vi "Test_AddMeas.vi"() -> ()   [LabVIEW 2019]
uses:
  ByteGSAPIBase.lvclass
panel:
  in  "ByteGSAPIBase in":refnum<class "ByteGSAPIBase.lvclass">
  out "ByteGSAPIBase out":refnum<class "ByteGSAPIBase.lvclass">
  out "Measurement_Id":i32
  out "error out":errorcluster
  in  "error in (no error)":errorcluster
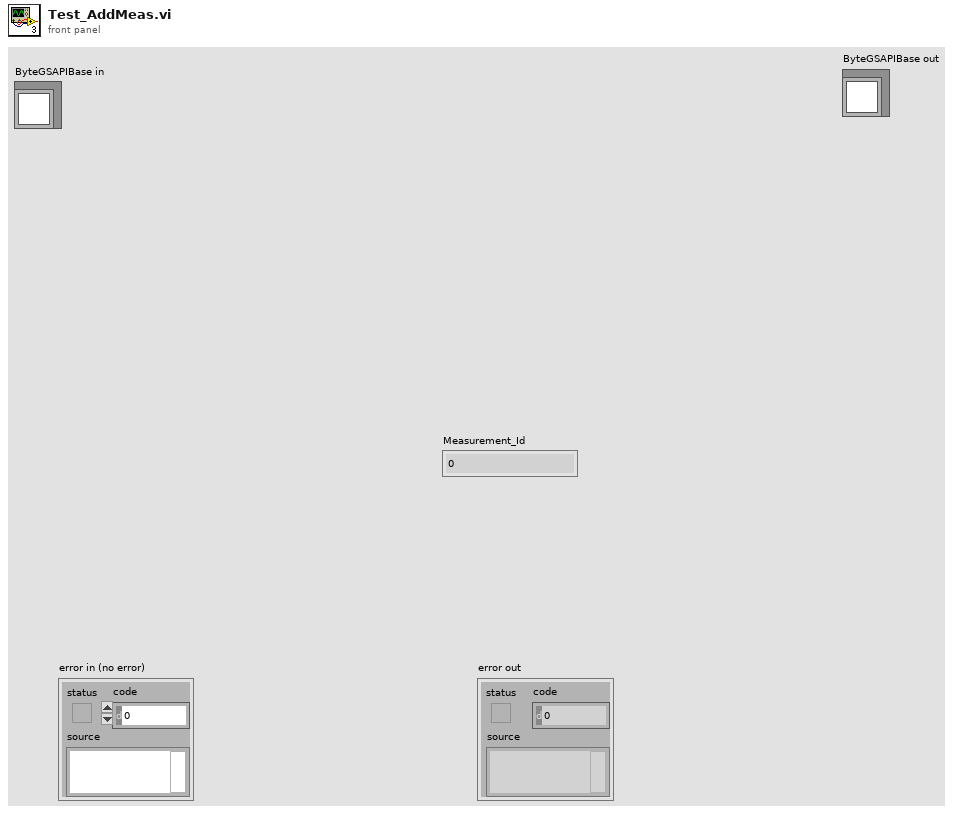
[diagram p1: front panel]
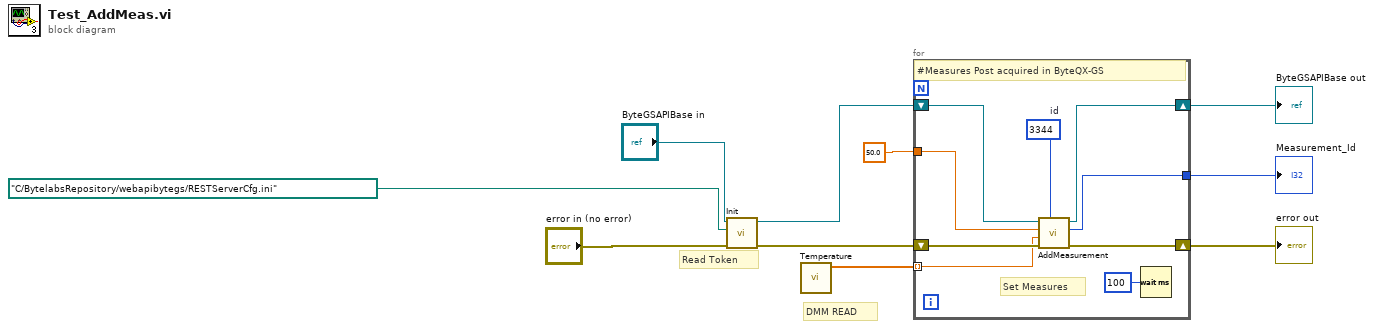
[diagram p0: block diagram]
diagram:
  # "Read Token"
  # "DMM READ"
  n1 = call-dynamic "Init.vi"("error in (no error)"="error in (no error)", "configuration file path"=path "C:/BytelabsRepository/webapibytegs/RESTServerCfg.ini", "ByteGSAPIBase in"="ByteGSAPIBase in") -> ("error out"=w6:errorcluster, "ByteGSAPIBase out"=w7:refnum<class "ByteGSAPIBase.lvclass">)  [unwired: 7 in]
  n2 = call "Temperature.vi"() -> ("Array"=w1:dbl[])  [unwired: 11 in]
  n3 = for {
    tunnel: [w16] -> w4
    shift-right: [w15] -> w3
    shift-left: w7 -> [w19]
    shift-right: [w17] -> w5
    shift-left: w6 -> [w18]
    tunnel: sgl 50.0 ("misura_riferimento") -> [w13]
    tunnel: w1 -> [w12] mode=indexing
    w14 = u16 3344  # id
    # "Set Measures"
    # "#Measures Post acquired in ByteQX-GS"
    n4 = call-dynamic "AddMeasurement.vi"("id"=w14, "error in (no error)"=w18, "misura_strumento"=w12, "misura_riferimento"=w13, "ByteGSAPIBase in"=w19) -> ("error out"=w17:errorcluster, "Measurement_Id"=w16:i32, "ByteGSAPIBase out"=w15:refnum<class "ByteGSAPIBase.lvclass">)  [unwired: 4 in]
    n5 = Wait (ms)(milliseconds to wait=u32 100) -> ()  [unwired: 1 out]
  }
  "error out" <- w5
  "Measurement_Id" <- w4
  "ByteGSAPIBase out" <- w3
